vi "AgPSA _Zero Span Single Point.vi"   [LabVIEW 2015]
uses:
  <instrlib>/Agilent MXA Series/Agilent MXA Series.lvlib
  <instrlib>/Agilent MXA Series/Public/Configure/Configure Frequency (Center Span).vi
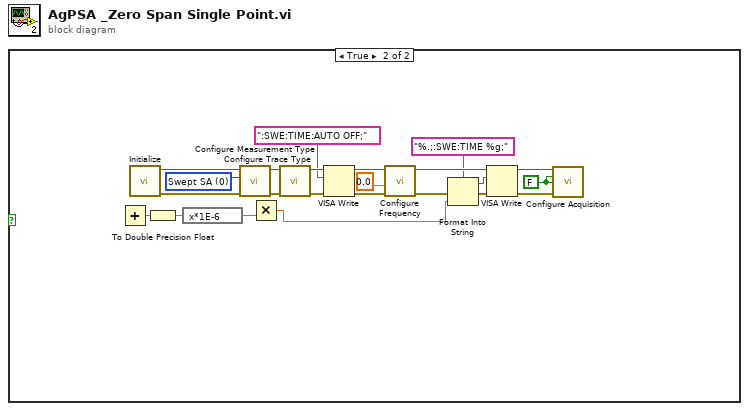
[diagram p0: block diagram]
diagram:
  n1 = case shown="True" {
    selector: _ -> [_ _]
    frame False {
    }
    frame True {
      w26 = 0 items=["Swept SA", "Channel Power", "Occupied Bandwidth", "Power Stat CCDF", "Adjacent Channel Power", "Burst Power", "Spurious Emissions", "Spectrum Emission Mask", "List Sweep"] ("Measurement Type")
      w10 = FALSE ("Auto Detector")
      n2 = Add() -> (x+y=w11:dbl)  [unwired: 2 in]
      n3 = call <instrlib>:"Initialize.vi"() -> ("error out"=w2:errorcluster, "VISA resource name out"=w14:refnum<visa-resource-name>)  [unwired: 10 in]
      n4 = To Double Precision Float(number=w11) -> (double precision float=w12:dbl)
      n5 = expression code="x*1E-6" ("us to s")(w12) -> (w5:dbl)
      n6 = call <instrlib>:"Configure Measurement Type.vi"("error in (no error)"=w2, "Measurement Type (0: Swept SA)"=w26, "VISA resource name"=w14) -> ("error out"=w23:errorcluster, "VISA resource name out"=w22:refnum<visa-resource-name>)  [unwired: 7 in]
      n7 = Multiply(y=w5) -> (x=w4:dbl, x*y=w3:dbl)
      n8 = call <instrlib>:"Configure Trace Type.vi"("error in (no error)"=w23, "VISA resource name"=w22) -> ("error out"=w17:errorcluster, "VISA resource name out"=w20:refnum<visa-resource-name>)  [unwired: 8 in]
      n9 = VISA Write(VISA resource name=w20, write buffer=":SWE:TIME:AUTO OFF;", error in (no error)=w17) -> (VISA resource name out=w19:refnum<visa-resource-name>, error out=w16:errorcluster)  [unwired: 1 out]
      n10 = call-poly <instrlib>:"Configure Frequency.vi"("error in (no error)"=w16, "Span (2.65E+10 Hz)"=0.0, "VISA resource name"=w19) -> ("error out"=w6:errorcluster, "VISA resource name out"=w15:refnum<visa-resource-name>, "Center Frequency (1.325E+10 Hz)"=w8:dbl)  [unwired: 6 in]
      n11 = Format Into String(format string="%.;:SWE:TIME %g;", error in=w6, w3) -> (resulting string=w1:string, error out=w7:errorcluster)  [unwired: 1 in]
      n12 = VISA Write(VISA resource name=w15, write buffer=w1, error in (no error)=w7) -> (VISA resource name out=w25:refnum<visa-resource-name>, error out=w21:errorcluster)  [unwired: 1 out]
      n13 = call <instrlib>:"Configure Acquisition.vi"("VISA resource name"=w25, "Enable Continuous Sweep (T: Enable)"=w10, "Auto Detector (T: Enable)"=w10, "error in (no error)"=w21) -> ("Sweep Points (1001)"=w9:i32)  [unwired: 9 in, 2 out]
    }
  }
